vi "GetFrontPanel.vi"(8 "Error In":errorcluster, 11 "reference in":refnum<class "TAFBaseGUI.lvclass">) -> (0 "Error Out":errorcluster, 2 "FrontPanelControl":refnum<class "FrontPanelControl.lvclass">, 3 "reference out":refnum<class "TAFBaseGUI.lvclass">)   [LabVIEW 2021, in "TAFBaseGUI.lvclass"]
uses:
  TAFBaseGUI.lvclass
  Library_UserInterface_FrontPanelControl/FrontPanelControl/FrontPanelControl.lvclass
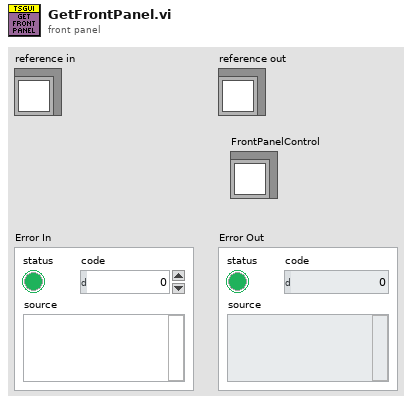
[diagram p1: front panel]
types:
  T1 = typedef "TAFBaseGUI.lvclass/ObjectAttributes.ctl" = cluster{"Name":string, "FPVIRef":refnum<vi>}
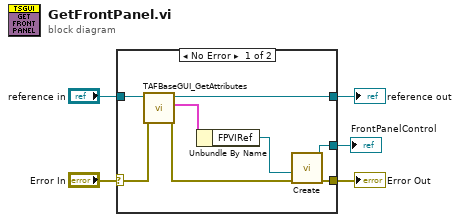
[diagram p0: block diagram]
diagram:
  n1 = case shown="No Error" "Error In" {
    selector: "Error In" -> [w13 w15]
    tunnel: [w8 w15] -> w4
    tunnel: [w9 w14] -> w2
    tunnel: "reference in" -> [w10 w14]
    tunnel: [w6 _] -> w1
    frame No Error {
      n2 = call "TAFBaseGUI_GetAttributes.vi"("error in (no error)"=w13, "reference in"=w10) -> ("error out"=w11:errorcluster, "Data"=w12:T1, "reference out"=w9:refnum<class "TAFBaseGUI.lvclass">)  [unwired: 6 in, 1 out]
      n3 = Unbundle By Name(w12) -> ("FPVIRef"=w7:refnum<vi>)
      n4 = call "Create.vi"("Error In"=w11, "VIRef"=w7) -> ("Error Out"=w8:errorcluster, "object out"=w6:refnum<class "FrontPanelControl.lvclass">)  [unwired: 8 in]
    }
    frame Error {
    }
  }
  "Error Out" <- w4
  "reference out" <- w2
  "FrontPanelControl" <- w1
